vi "생산자소비자.vi"() -> ()   [LabVIEW 2014]
uses:
  <vilib>/Analysis/NI_AALBase.lvlib
panel:
  out "웨이브폼 그래프":dbl[](graph)
  in  "확인 버튼":bool
  in  "정지":bool
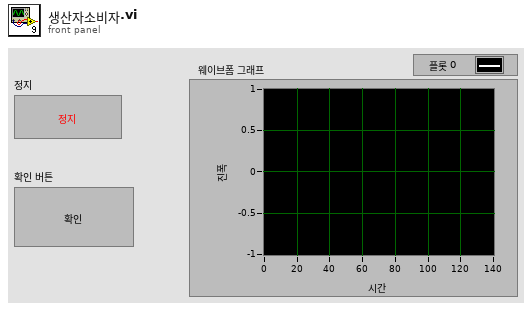
[diagram p1: front panel]
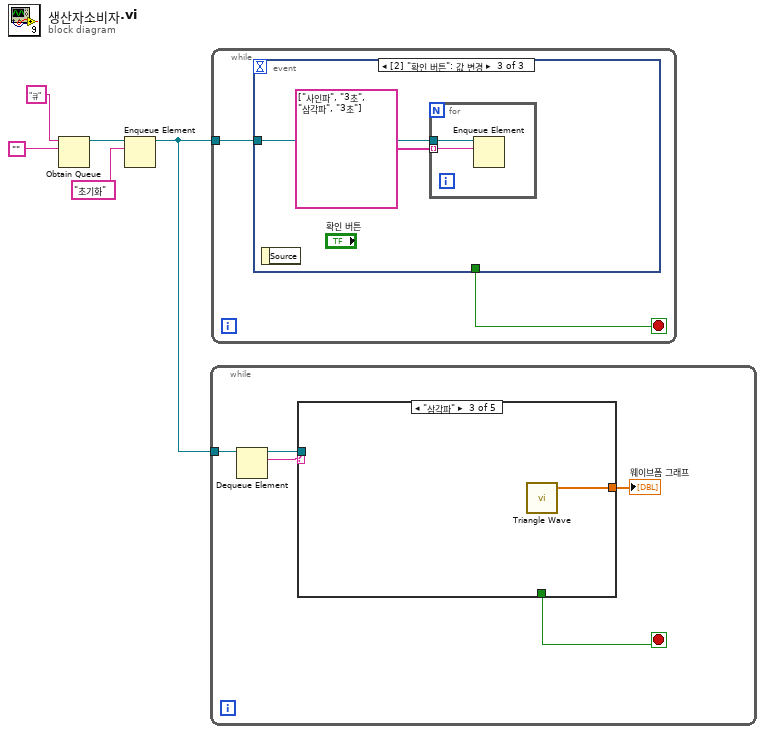
[diagram p0: block diagram]
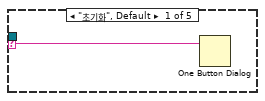
[diagram p2: hidden frame]
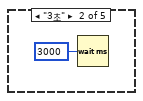
[diagram p3: hidden frame]
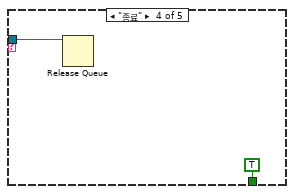
[diagram p4: hidden frame]
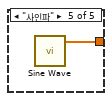
[diagram p5: hidden frame]
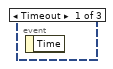
[diagram p6: hidden frame]
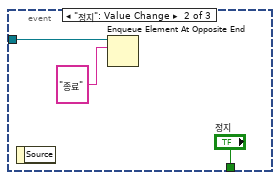
[diagram p7: hidden frame]
diagram:
  n1 = Obtain Queue(name (unnamed)="큐" ("이름(이름없음)"), element data type="") -> (queue out=w5:refnum<queue>)  [unwired: 3 in, 2 out]
  n2 = Enqueue Element(queue=w5, element="초기화" ("원소")) -> (queue out=w1:refnum<queue>)  [unwired: 2 in, 2 out]
  n3 = while {
    tunnel: w1 -> [w10]
    stop <- w7 stop-if-true
    n4 = Dequeue Element(queue=w10) -> (queue out=w6:refnum<queue>, element=w9:string)  [unwired: 2 in, 2 out]
    n5 = case shown="\"삼각파\"" w9 {
      selector: w9 -> [w11 _ _ _ _]
      tunnel: [_ _ _ TRUE _] -> w7
      tunnel: [_ _ w13 _ w16] -> w8
      tunnel: w6 -> [_ _ _ w14 _]
      frame "초기화", Default {
        n6 = One Button Dialog(message=w11) -> ()  [unwired: 1 in, 1 out]
      }
      frame "3초" {
        n7 = Wait (ms)(milliseconds to wait=u32 3000 ("대기 시간(ms)")) -> ()  [unwired: 1 out]
      }
      frame "삼각파" {
        n8 = call <vilib>:"Triangle Wave.vi"() -> ("triangle wave"=w13:dbl[])  [unwired: 5 in, 2 out]
      }
      frame "종료" {
        n9 = Release Queue(queue=w14) -> ()  [unwired: 2 in, 3 out]
      }
      frame "사인파" {
        n10 = call <vilib>:"Sine Wave.vi"() -> ("sine wave"=w16:dbl[])  [unwired: 5 in, 2 out]
      }
    }
    "웨이브폼 그래프" <- w8
  }
  n11 = while {
    tunnel: w1 -> [w18]
    stop <- w17 stop-if-true
    n12 = event shown="[2] \"확인 버튼\": 값 변경" {
      selector: _ -> [_ _ _]
      dyn-events: _ -> [_ _ _]
      timeout: _ -> [_ _ _]
      tunnel: w18 -> [_ w21 w23]
      tunnel: [_ "정지" _] -> w17
      event Timeout {
        n13 = event-data() -> ()  [unwired: 1 in, 1 out]
      }
      event "정지": Value Change {
        n14 = event-data() -> ()  [unwired: 1 in, 1 out]
        n15 = Enqueue Element At Opposite End(queue=w21, element="종료" ("원소")) -> ()  [unwired: 2 in, 3 out]
      }
      event "확인 버튼": Value Change {
        n16 = event-data() -> ()  [unwired: 1 in, 1 out]
        n17 = for {
          tunnel: w23 -> [w25]
          tunnel: string[] ["사인파", "3초", "삼각파", "3초"] -> [w24] mode=indexing
          n18 = Enqueue Element(queue=w25, element=w24) -> ()  [unwired: 2 in, 3 out]
        }
      }
    }
  }
